vi "Make persistent.vi"(8 "error in (no error)":errorcluster, 11 "PS Control Persistence Actor in":refnum<class "PS Control Persistence Actor.lvclass">) -> (0 "error out":errorcluster, 3 "PS Control Persistence Actor out":refnum<class "PS Control Persistence Actor.lvclass">)   [LabVIEW 2025, in "PS Control Persistence.lvlib" / "PS Control Persistence Actor.lvclass"]
doc: "Author: Scott Hannahs <sth@magnet.fsu.edu>\n\nThis software is licensed for use under the “MIT License\"\nCopyright (c) 2025 Scott Hannahs, sth@sth@magnet.sthnet.net\n\nPermission is hereby granted, free of charge, to any person obtaining a copy of this software and associated documentation files (the \"Software\"), to deal in the Software without restriction, including without limitation the rights to use, copy, modify, merge, publish, distribute, sublicense, and/or sell copies of the Software, and to permit persons to whom the Software is furnished to do so, subject to the following conditions: The above copyright notice and this permission notice shall be included in all copies or substantial portions of the Software.\n\nTHE SOFTWARE IS PROVIDED \"AS IS\", WITHOUT WARRANTY OF ANY KIND, EXPRESS OR IMPLIED, INCLUDING BUT NOT LIMITED TO THE WARRANTIES OF MERCHANTABILITY, FITNESS FOR A PARTICULAR PURPOSE AND NONINFRINGEMENT. IN NO EVENT SHALL THE AUTHORS OR COPYRIGHT HOLDERS BE LIABLE FOR ANY CLAIM, DAMAGES OR OTHER LIABILITY, WHETHER IN AN ACTION OF CONTRACT, TORT OR OTHERWISE, ARISING FROM, OUT OF OR IN CONNECTION WITH THE SOFTWARE OR THE USE OR OTHER DEALINGS IN THE SOFTWARE."
uses:
  PS Control Persistence Actor.lvclass
  PS Driver/PS Driver with Persistence.lvclass
  PS Control Actor.lvclass/PS Control Actor.ctl
  PS Control Actor.lvclass
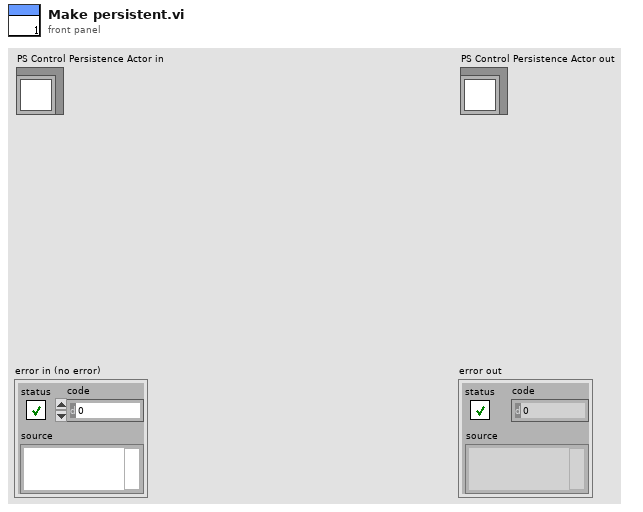
[diagram p1: front panel]
types:
  T1 = enum8{"Enabled", "Disabled", "Disabled and Grayed Out"}
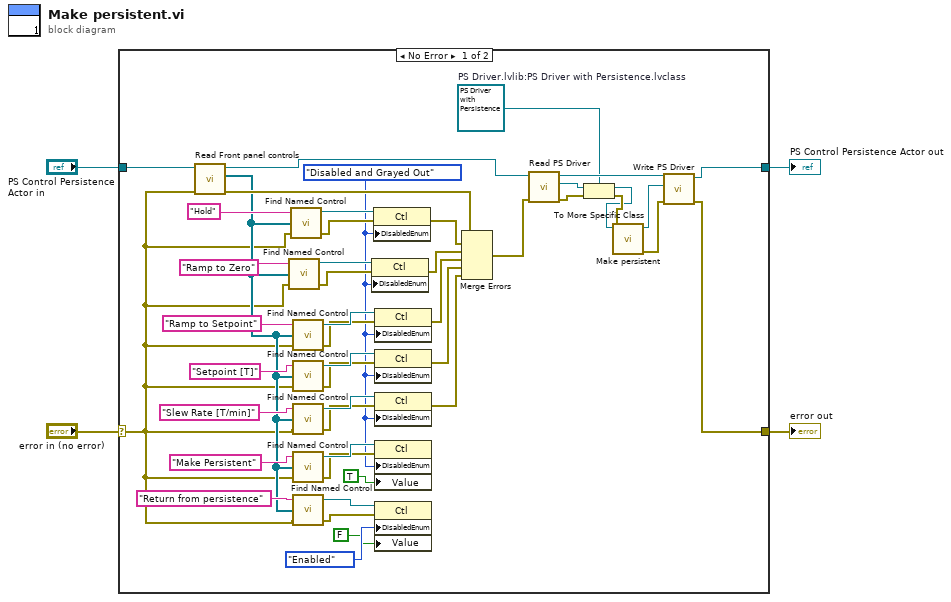
[diagram p0: block diagram]
diagram:
  n1 = case shown="No Error" "error in (no error)" {
    selector: "error in (no error)" -> [w9 w52]
    tunnel: [w25 w52] -> w3
    tunnel: [w26 w51] -> w1
    tunnel: "PS Control Persistence Actor in" -> [w38 w51]
    frame No Error {
      w17 = refnum<class "PS Driver with Persistence.lvclass"> refnum  # PS Driver.lvlib:PS Driver with Persistence.lvclass
      w8 = T1."Disabled and Grayed Out" ("Disabled")
      n2 = call "Read Front panel controls.vi"("error in (no error)"=w9, "PS Control Actor in"=w38) -> ("error out"=w37:errorcluster, "Front panel controls"=w10:refnum<vi>[], "PS Control Actor out"=w28:refnum<class "PS Control Persistence Actor.lvclass">)  [unwired: 7 in]
      n3 = call "Find Named Control.vi"("error in"=w9, "All Controls"=w10, "Control Name"="Ramp to Zero") -> ("error out"=w46:errorcluster, "Ctl Refnum"=w47:refnum<vi>)  [unwired: 1 out]
      n4 = call "Find Named Control.vi"("error in"=w9, "All Controls"=w10, "Control Name"="Hold") -> ("error out"=w49:errorcluster, "Ctl Refnum"=w50:refnum<vi>)  [unwired: 1 out]
      n5 = call "Find Named Control.vi"("error in"=w9, "All Controls"=w10, "Control Name"="Ramp to Setpoint") -> ("error out"=w41:errorcluster, "Ctl Refnum"=w42:refnum<vi>)  [unwired: 1 out]
      n6 = call "Find Named Control.vi"("error in"=w9, "All Controls"=w10, "Control Name"="Setpoint [T]") -> ("error out"=w35:errorcluster, "Ctl Refnum"=w36:refnum<vi>)  [unwired: 1 out]
      n7 = call "Find Named Control.vi"("error in"=w9, "All Controls"=w10, "Control Name"="Slew Rate [T/min]") -> ("error out"=w33:errorcluster, "Ctl Refnum"=w34:refnum<vi>)  [unwired: 1 out]
      n8 = call "Find Named Control.vi"("error in"=w9, "All Controls"=w10, "Control Name"="Make Persistent") -> ("error out"=w15:errorcluster, "Ctl Refnum"=w16:refnum<vi>)  [unwired: 1 out]
      n9 = call "Find Named Control.vi"("error in"=w9, "All Controls"=w10, "Control Name"="Return from persistence") -> ("error out"=w13:errorcluster, "Ctl Refnum"=w14:refnum<vi>)  [unwired: 1 out]
      n10 = property class="Ctl"(reference=w47, error in=w46, "DisabledEnum"=w8) -> (error out=w43:errorcluster)  [unwired: 1 out]
      n11 = property class="Ctl"(reference=w50, error in=w49, "DisabledEnum"=w8) -> (error out=w44:errorcluster)  [unwired: 1 out]
      n12 = property class="Ctl"(reference=w42, error in=w41, "DisabledEnum"=w8) -> (error out=w39:errorcluster)  [unwired: 1 out]
      n13 = property class="Ctl"(reference=w36, error in=w35, "DisabledEnum"=w8) -> (error out=w30:errorcluster)  [unwired: 1 out]
      n14 = property class="Ctl"(reference=w34, error in=w33, "DisabledEnum"=w8) -> (error out=w29:errorcluster)  [unwired: 1 out]
      n15 = property class="Ctl"(reference=w16, error in=w15, "DisabledEnum"=w8, "Value"=TRUE) -> ()  [unwired: 2 out]
      n16 = property class="Ctl"(reference=w14, error in=w13, "DisabledEnum"=T1."Enabled" ("Disabled"), "Value"=FALSE) -> ()  [unwired: 2 out]
      n17 = Merge Errors(w37, w44, w43, w39, w30, w29) -> (w23:errorcluster)
      n18 = call-dynamic "Read PS Driver.vi"("error in (no error)"=w23, "PS Control Persistence Actor in"=w28) -> ("error out"=w21:errorcluster, "PS Driver.lvlib:PS Driver.lvclass"=w20:refnum<class "PS Driver.lvclass">, "PS Control Persistence Actor out"=w27:refnum<class "PS Control Persistence Actor.lvclass">)  [unwired: 7 in]
      n19 = To More Specific Class(target class=w17, reference=w20, error in=w21) -> (specific class reference=w18:refnum<class "PS Driver with Persistence.lvclass">, error out=w19:errorcluster)
      n20 = call-dynamic "Make persistent.vi"("error in (no error)"=w19, "PS Driver with Persistence in"=w18) -> ("error out"=w24:errorcluster, "PS Driver with Persistence out"=w22:refnum<class "PS Driver with Persistence.lvclass">)  [unwired: 8 in]
      n21 = call-dynamic "Write PS Driver.vi"("error in (no error)"=w24, "PS Driver.lvlib:PS Driver.lvclass"=w22, "PS Control Persistence Actor in"=w27) -> ("error out"=w25:errorcluster, "PS Control Persistence Actor out"=w26:refnum<class "PS Control Persistence Actor.lvclass">)  [unwired: 7 in]
    }
    frame Error {
    }
  }
  "error out" <- w3
  "PS Control Persistence Actor out" <- w1
